vi "ULx Create IOTask.vi"(8 "error in":errorcluster, 10 "taskType":i32(ring) items=["AnalogInput", "AnalogOutput", "DigitalInput", "DigitalOutput", "CounterInput", "CounterOutput", "CompositeInput", "CompositeOutput", "TemperatureInput"], 11 "i/o task in":refnum<k24>) -> (0 "error out":errorcluster, 3 "i/o task out":refnum<k24>)   [LabVIEW 2020]
uses:
  C:/Users/William/Documents/LV 2020 builds/LeaktestDAQ/Source-v33/ULx_LV.dll
  ULx_LV.dll
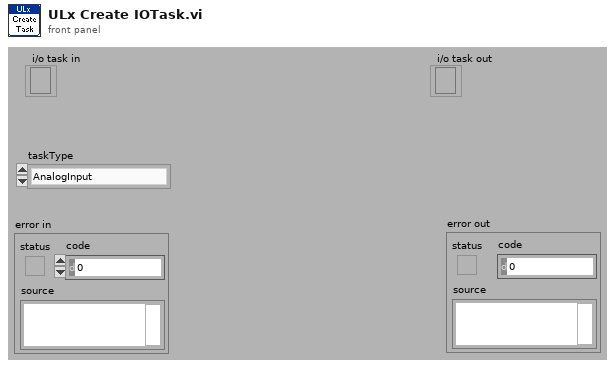
[diagram p1: front panel]
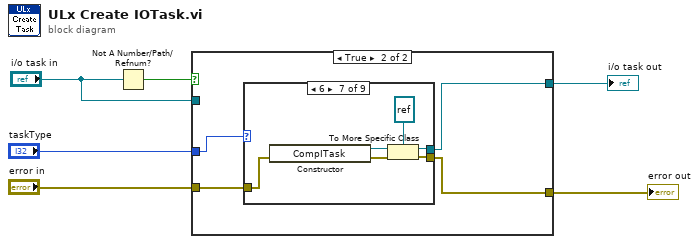
[diagram p0: block diagram]
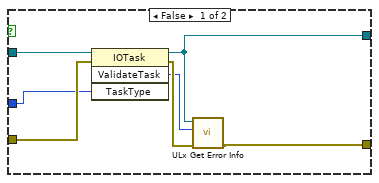
[diagram p2: hidden frame]
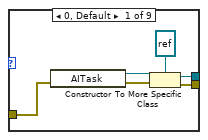
[diagram p3: hidden frame]
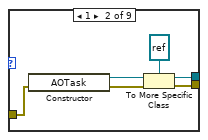
[diagram p4: hidden frame]
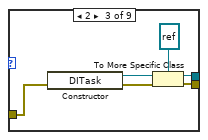
[diagram p5: hidden frame]
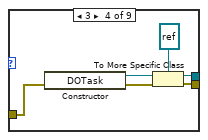
[diagram p6: hidden frame]
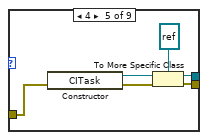
[diagram p7: hidden frame]
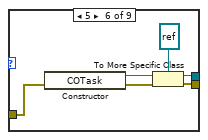
[diagram p8: hidden frame]
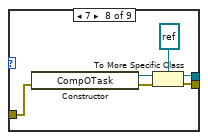
[diagram p9: hidden frame]
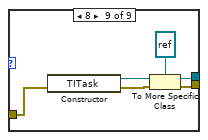
[diagram p10: hidden frame]
diagram:
  n1 = Not A Number/Path/Refnum?(number/path/refnum="i/o task in") -> (NaN/Path/Refnum?=w6:bool)
  n2 = case shown="True" w6 {
    tunnel: "taskType" -> [w11 w16]
    tunnel: [w8 w15] -> w2
    tunnel: "i/o task in" -> [w13 _]
    tunnel: "error in" -> [w12 w17]
    tunnel: [w7 w14] -> w1
    frame False {
      n3 = invoke class="IOTask" method="ValidateTask"(reference=w13, error in=w12, "TaskType"=w11) -> (reference out=w8:refnum<k24>, error out=w10:errorcluster, "ValidateTask"=w9:i32)  [unwired: 1 in, 1 out]
      n4 = call "ULx Get Error Info.vi"("error in"=w10, "ErrorCode"=w9, "task in"=w8) -> ("error out"=w7:errorcluster)  [unwired: 8 in]
    }
    frame True {
      n5 = case shown="6" w16 {
        tunnel: w17 -> [w23 w29 w35 w41 w47 w53 w59 w65 w71]
        tunnel: [w19 w25 w31 w37 w43 w49 w55 w61 w68] -> w15
        tunnel: [w18 w24 w30 w36 w42 w48 w54 w60 w66] -> w14
        frame 0, Default {
          n6 = constructor class="AITask"(error in=w23) -> (reference out=w22:refnum<k24>, error out=w21:errorcluster)  [unwired: 2 in, 1 out]
          n7 = To More Specific Class(target class=refnum<k24> refnum, reference=w22, error in=w21) -> (specific class reference=w19:refnum<k24>, error out=w18:errorcluster)
        }
        frame 1 {
          n8 = constructor class="AOTask"(error in=w29) -> (reference out=w28:refnum<k24>, error out=w27:errorcluster)  [unwired: 2 in, 1 out]
          n9 = To More Specific Class(target class=refnum<k24> refnum, reference=w28, error in=w27) -> (specific class reference=w25:refnum<k24>, error out=w24:errorcluster)
        }
        frame 2 {
          n10 = constructor class="DITask"(error in=w35) -> (reference out=w33:refnum<k24>, error out=w34:errorcluster)  [unwired: 2 in, 1 out]
          n11 = To More Specific Class(target class=refnum<k24> refnum, reference=w33, error in=w34) -> (specific class reference=w31:refnum<k24>, error out=w30:errorcluster)
        }
        frame 3 {
          n12 = constructor class="DOTask"(error in=w41) -> (reference out=w39:refnum<k24>, error out=w40:errorcluster)  [unwired: 2 in, 1 out]
          n13 = To More Specific Class(target class=refnum<k24> refnum, reference=w39, error in=w40) -> (specific class reference=w37:refnum<k24>, error out=w36:errorcluster)
        }
        frame 4 {
          n14 = constructor class="CITask"(error in=w47) -> (reference out=w45:refnum<k24>, error out=w46:errorcluster)  [unwired: 2 in, 1 out]
          n15 = To More Specific Class(target class=refnum<k24> refnum, reference=w45, error in=w46) -> (specific class reference=w43:refnum<k24>, error out=w42:errorcluster)
        }
        frame 5 {
          n16 = constructor class="COTask"(error in=w53) -> (reference out=w51:refnum<k24>, error out=w52:errorcluster)  [unwired: 2 in, 1 out]
          n17 = To More Specific Class(target class=refnum<k24> refnum, reference=w51, error in=w52) -> (specific class reference=w49:refnum<k24>, error out=w48:errorcluster)
        }
        frame 6 {
          n18 = constructor class="CompITask"(error in=w59) -> (reference out=w57:refnum<k24>, error out=w58:errorcluster)  [unwired: 2 in, 1 out]
          n19 = To More Specific Class(target class=refnum<k24> refnum, reference=w57, error in=w58) -> (specific class reference=w55:refnum<k24>, error out=w54:errorcluster)
        }
        frame 7 {
          n20 = constructor class="CompOTask"(error in=w65) -> (reference out=w63:refnum<k24>, error out=w64:errorcluster)  [unwired: 2 in, 1 out]
          n21 = To More Specific Class(target class=refnum<k24> refnum, reference=w63, error in=w64) -> (specific class reference=w61:refnum<k24>, error out=w60:errorcluster)
        }
        frame 8 {
          n22 = constructor class="TITask"(error in=w71) -> (reference out=w69:refnum<k24>, error out=w67:errorcluster)  [unwired: 2 in, 1 out]
          n23 = To More Specific Class(target class=refnum<k24> refnum, reference=w69, error in=w67) -> (specific class reference=w68:refnum<k24>, error out=w66:errorcluster)
        }
      }
    }
  }
  "i/o task out" <- w2
  "error out" <- w1
